vi "Set Panel Initial State.vi"(10 "Title":string, 11 "Main Vi Ref":refnum<vi>) -> (0 "error out":errorcluster)   [LabVIEW 2019, in "Panther Dashboard.lvlib"]
uses:
  Panther Dashboard.lvlib
  Shared/Shared.lvlib
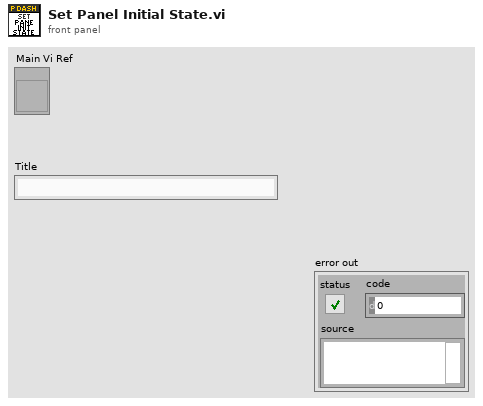
[diagram p1: front panel]
types:
  T1 = enum32{"Invalid", "Standard", "Closed", "Hidden", "Minimized", "Maximized"}
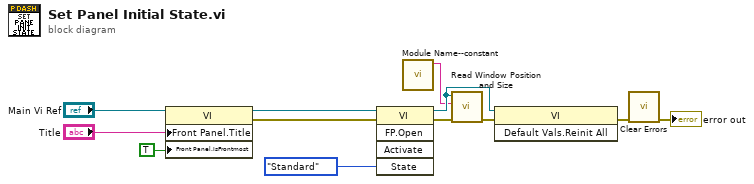
[diagram p0: block diagram]
diagram:
  n1 = property on="Property Node" class="VI"(reference="Main Vi Ref", "Front Panel.Title"="Title", "Front Panel.IsFrontmost"=TRUE ("Front Panel Window:Is Frontmost")) -> (reference out=w4:refnum<vi>, error out=w11:errorcluster)  [unwired: 1 in]
  n2 = invoke on="Invoke Node" class="VI" method="FP.Open"(reference=w4, error in=w11, "State"=T1."Standard") -> (reference out=w2:refnum<vi>, error out=w12:errorcluster)  [unwired: 2 in, 3 out]
  n3 = call "Module Name--constant.vi"() -> ("Module Name"=w1:string)  [unwired: 11 in]
  n4 = call "Read Window Position and Size.vi"("error in"=w12, "Position Key"=w1, "VI Refnum"=w2) -> ("error out"=w8:errorcluster)  [unwired: 8 in]
  n5 = invoke class="VI" method="Default Vals.Reinit All"(reference=w2, error in=w8) -> (error out=w10:errorcluster)  [unwired: 1 in, 2 out]
  n6 = call <vilib>:"Clear Errors.vi"("error in (no error)"=w10) -> ("error out"=→"error out":errorcluster)  [unwired: 5 in, 1 out]
